vi "Run Script.vi"(8 "error in (no error)":errorcluster caption="错误输入（无错误）", 11 "虚拟 输入":refnum<class "虚拟.lvclass">) -> (0 "error out":errorcluster caption="错误输出", 3 "虚拟 输出":refnum<class "虚拟.lvclass">)   [LabVIEW 2020, in "虚拟.lvclass"]
uses:
  <vilib>/Analysis/NI_AALBase.lvlib
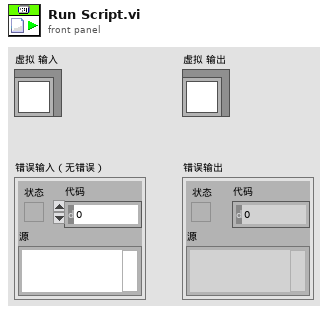
[diagram p1: front panel]
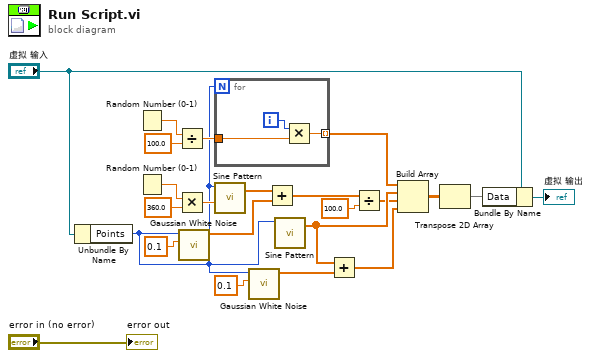
[diagram p0: block diagram]
diagram:
  n1 = Unbundle By Name("虚拟 输入") -> ("Points"=w3:i32)
  n2 = Random Number (0-1)() -> (number: 0 to 1=w12:dbl)
  n3 = Random Number (0-1)() -> (number: 0 to 1=w10:dbl)
  n4 = Divide(x=w12, y=100.0) -> (x/y=w13:dbl)
  n5 = Multiply(x=w10, y=360.0) -> (x*y=w8:dbl)
  n6 = call <vilib>:"Gaussian White Noise.vi"("standard deviation"=0.1, "samples"=w3) -> ("Gaussian noise pattern"=w17:dbl[])  [unwired: 8 in, 1 out]
  n7 = for {
    N: w3 -> [_]
    tunnel: [w25] -> w20 mode=indexing
    tunnel: w13 -> [w24]
    i -> [w26]
    n8 = Multiply(x=w26, y=w24) -> (x*y=w25:dbl)
  }
  n9 = call <vilib>:"Sine Pattern.vi"("phase(degrees)"=w8, "samples"=w3) -> ("Sinusoidal Pattern"=w21:dbl[])  [unwired: 2 in, 1 out]
  n10 = call <vilib>:"Gaussian White Noise.vi"("standard deviation"=0.1, "samples"=w3) -> ("Gaussian noise pattern"=w14:dbl[])  [unwired: 8 in, 1 out]
  n11 = Add(x=w21, y=w17) -> (x+y=w18:dbl[])
  n12 = call <vilib>:"Sine Pattern.vi"("samples"=w3) -> ("Sinusoidal Pattern"=w7:dbl[])  [unwired: 3 in, 1 out]
  n13 = Add(x=w7, y=w14) -> (x+y=w16:dbl[])
  n14 = Divide(x=w18, y=100.0) -> (x/y=w6:dbl[])
  n15 = Build Array(w20, w7, w6, w16) -> (w5:dbl[][])
  n16 = Transpose 2D Array(2D array=w5) -> (transposed array=w1:dbl[][])
  n17 = Bundle By Name(cluster="虚拟 输入", "Data"=w1) -> (→"虚拟 输出":refnum<class "虚拟.lvclass">)
  "error out" <- "error in (no error)"
